vi "Update Position.vi"(2 "error in (no error)":errorcluster, 3 "Time Since Last Update":dbl, 4 "Car.lvclass":refnum<class "Car.lvclass">) -> (0 "error out":errorcluster, 1 "Car.lvclass 2":refnum<class "Car.lvclass">)   [LabVIEW 2015, in "Car.lvclass"]
uses:
  Car.lvclass
  Car.lvclass/Car.ctl
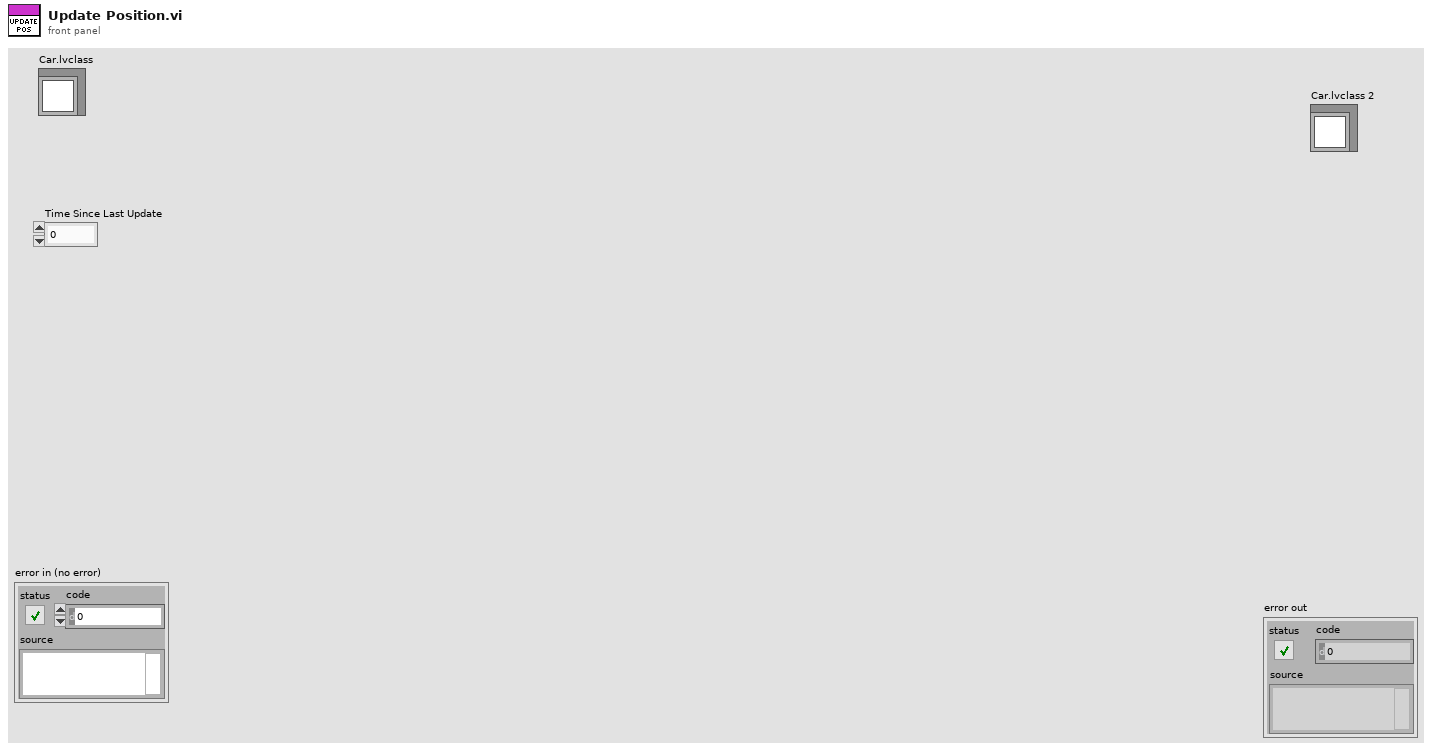
[diagram p1: front panel]
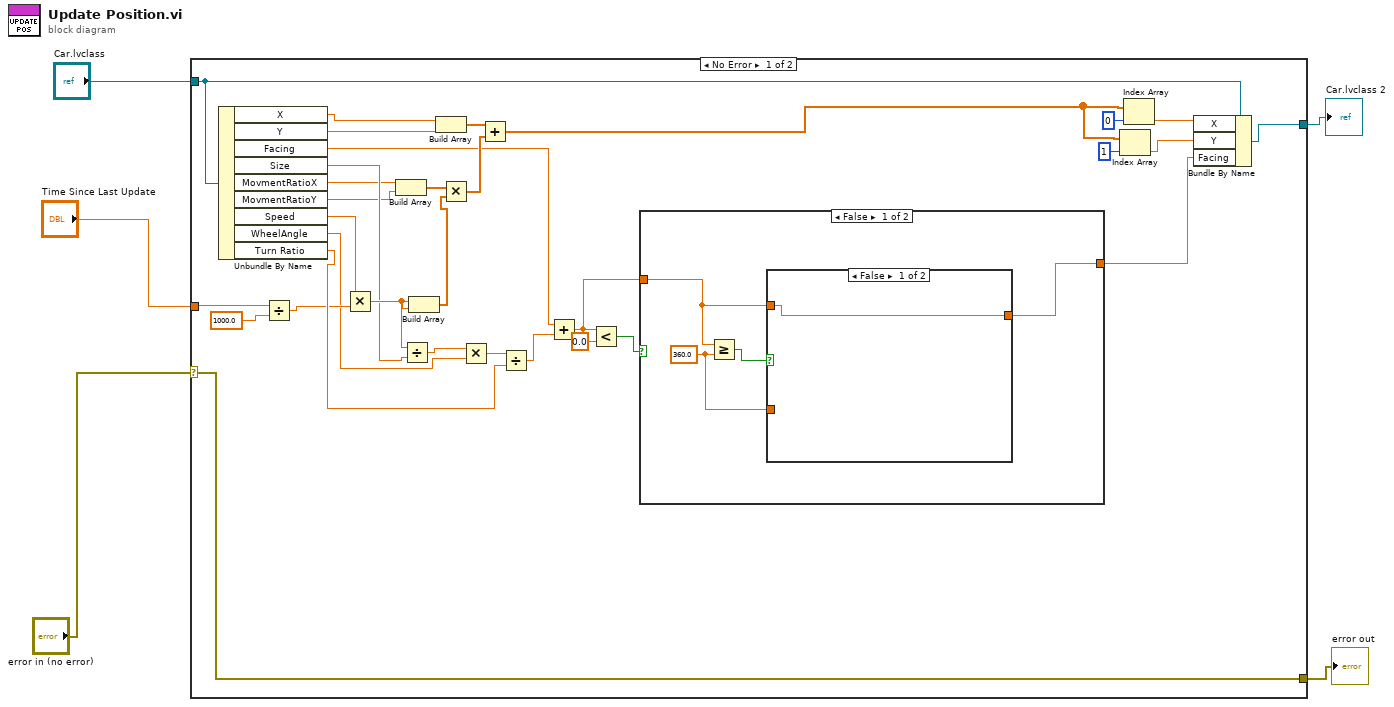
[diagram p0: block diagram]
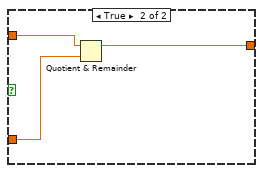
[diagram p2: hidden frame]
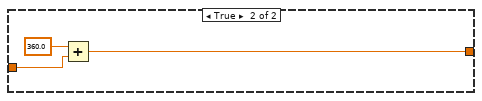
[diagram p3: hidden frame]
diagram:
  n1 = case shown="No Error" "error in (no error)" {
    selector: "error in (no error)" -> [w37 w50]
    tunnel: [w37 w50] -> w4
    tunnel: [w11 w49] -> w3
    tunnel: "Car.lvclass" -> [w23 w49]
    tunnel: "Time Since Last Update" -> [w10 _]
    frame No Error {
      n2 = Unbundle By Name(w23) -> ("X"=w27:dbl, "Y"=w26:dbl, "Facing"=w16:dbl, "Size"=w35:dbl, "MovmentRatioX"=w31:dbl, "MovmentRatioY"=w30:dbl, "Speed"=w7:dbl, "WheelAngle"=w6:dbl, "Turn Ratio"=w32:dbl)
      n3 = Divide(x=w10, y=1000.0) -> (x/y=w8:dbl)
      n4 = Multiply(x=w7, y=w8) -> (x*y=w36:dbl)
      n5 = Build Array(w31, w30) -> (w29:dbl[])
      n6 = Divide(x=w36, y=w35) -> (x/y=w34:dbl)
      n7 = Build Array(w36, w36) -> (w28:dbl[])
      n8 = Build Array(w27, w26) -> (w25:dbl[])
      n9 = Multiply(x=w29, y=w28) -> (x*y=w24:dbl[])
      n10 = Multiply(x=w34, y=w6) -> (x*y=w33:dbl)
      n11 = Add(x=w25, y=w24) -> (x+y=w18:dbl[])
      n12 = Divide(x=w33, y=w32) -> (x/y=w17:dbl)
      n13 = Add(x=w16, y=w17) -> (x+y=w13:dbl)
      n14 = Less?(x=w13, y=0.0) -> (x < y?=w14:bool)
      n15 = case shown="False" w14 {
        tunnel: w13 -> [w40 w47]
        tunnel: [w38 w46] -> w12
        frame False {
          w39 = 360.0 ("y")
          n16 = Greater Or Equal?(x=w40, y=w39) -> (x >= y?=w41:bool)
          n17 = case shown="False" w41 {
            tunnel: w40 -> [w42 w45]
            tunnel: w39 -> [_ w44]
            tunnel: [w42 w43] -> w38
            frame False {
            }
            frame True {
              n18 = Quotient & Remainder(x=w45, y=w44) -> (x-y*floor(x/y)=w43:dbl)  [unwired: 1 out]
            }
          }
        }
        frame True {
          n19 = Add(x=360.0, y=w47) -> (x+y=w46:dbl)
        }
      }
      n20 = Index Array(array=w18, index=1) -> (element=w20:dbl)
      n21 = Index Array(array=w18, index=0) -> (element=w19:dbl)
      n22 = Bundle By Name(cluster=w23, "X"=w19, "Y"=w20, "Facing"=w12) -> (w11:refnum<class "Car.lvclass">)
    }
    frame Error {
    }
  }
  "Car.lvclass 2" <- w3
  "error out" <- w4
